vi "find start.vi"(6 "pulse sample":i32=5, 8 "trama length":i32=80, 9 "level":dbl=0.1 format="%#_13g", 10 "Trigger found in":bool, 11 "signal in":dbl[](array[numeric])) -> (2 "Trigger found":bool, 3 "signal out":dbl[](array[numeric]))   [LabVIEW 2017]
uses:
  <vilib>/Analysis/baseanly.llb/Real Dot Product.vi
  <vilib>/Analysis/NI_AAL_SigProc.lvlib
  <vilib>/Analysis/NI_AALBase.lvlib
panel:
  out "Numeric":dbl
  out "max index(es)":i32
  out "Waveform Graph":dbl[](graph)
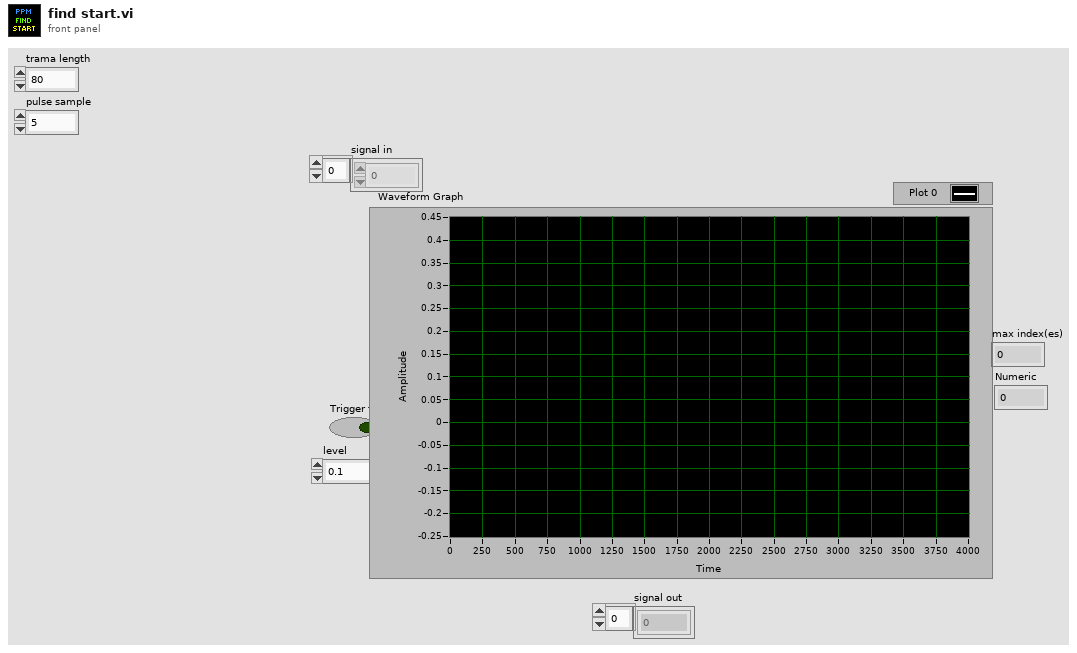
[diagram p1: front panel]
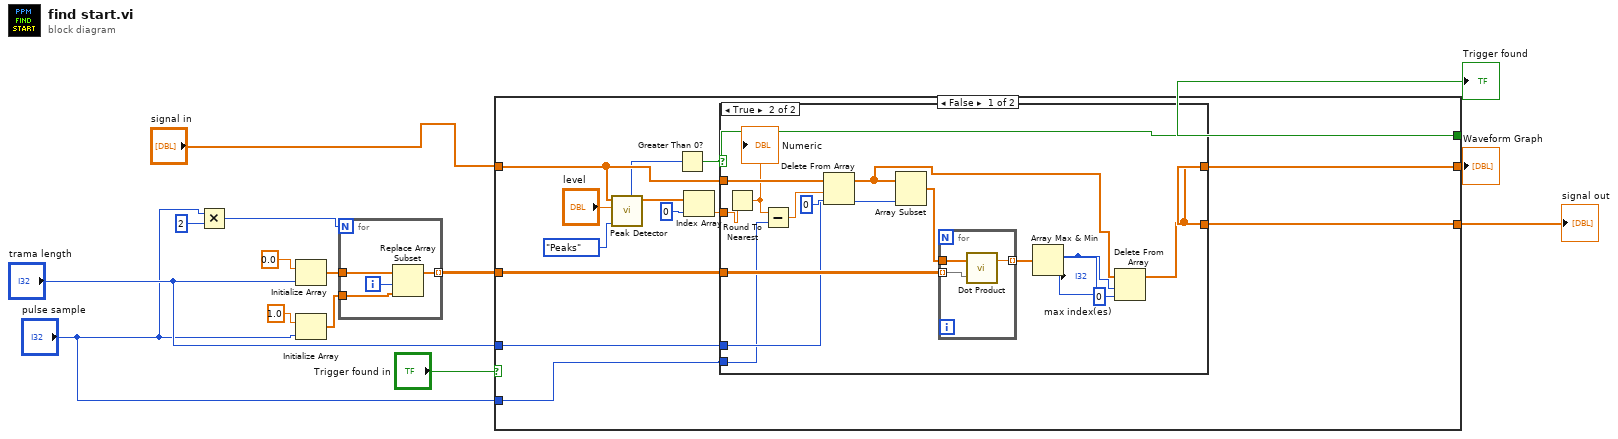
[diagram p0: block diagram]
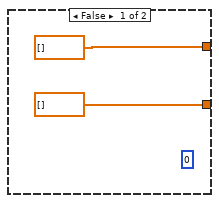
[diagram p2: hidden frame]
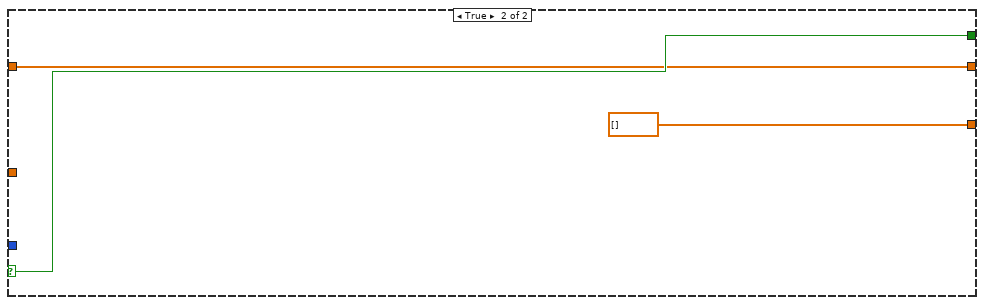
[diagram p3: hidden frame]
diagram:
  n1 = Multiply(x="pulse sample", y=u8 2) -> (x*y=w2:i32)
  n2 = Initialize Array(0.0 ("element"), "trama length") -> (w9:dbl[])
  n3 = Initialize Array(1.0 ("element"), "pulse sample") -> (w7:dbl[])
  n4 = for {
    N: w2 -> [_]
    tunnel: w9 -> [w17]
    tunnel: w7 -> [w16]
    tunnel: [w14] -> w6 mode=indexing
    i -> [w15]
    n5 = Replace Array Subset(array=w17, new element=w16, index=w15) -> (w14:dbl[])
  }
  n6 = case shown="False" "Trigger found in" {
    selector: "Trigger found in" -> [_ w52]
    tunnel: [w27 w52] -> w13
    tunnel: [w30 w51] -> w11
    tunnel: "signal in" -> [w28 w51]
    tunnel: [w20 dbl[] [] ("signal in")] -> _
    tunnel: w6 -> [w21 _]
    tunnel: "trama length" -> [w19 _]
    tunnel: "pulse sample" -> [w18 _]
    frame False {
      n7 = call <vilib>:"Peak Detector.vi"("peaks/valleys"=enum32{"Peaks", "Valleys"}."Peaks", "threshold"="level", "X"=w28) -> ("Locations"=w24:dbl[], "# found"=w26:i32)  [unwired: 4 in, 3 out]
      n8 = Greater Than 0?(x=w26) -> (x > 0?=w27:bool)
      n9 = Index Array(array=w24, index=0) -> (element=w23:dbl)
      n10 = case shown="True" w27 {
        tunnel: w28 -> [_ w46]
        tunnel: [dbl[] [] ("Y") w38] -> w30
        tunnel: w23 -> [_ w37]
        tunnel: [dbl[] [] ("signal in") w38] -> w20
        tunnel: w21 -> [_ w41]
        tunnel: w19 -> [_ w34]
        tunnel: w18 -> [_ w33]
        frame False {
          (unwired) 0
        }
        frame True {
          n11 = Round To Nearest(number=w37) -> (nearest integer value=w36:dbl)
          "Numeric" <- w36
          n12 = Subtract(x=w36, y=w33) -> (x-y=w44:dbl)
          n13 = Delete From Array(array=w46, length=w44, index=0) -> (array with subset deleted=w35:dbl[])  [unwired: 1 out]
          n14 = Array Subset(array=w35, length=w34) -> (w43:dbl[])  [unwired: 1 in]
          n15 = for {
            tunnel: w43 -> [w49]
            tunnel: [w48] -> w42 mode=indexing
            tunnel: w41 -> [w47] mode=indexing
            n16 = call-poly <vilib>:"Dot Product.vi"("Y Vector"=w47, "X Vector"=w49) -> ("X * Y"=w48:dbl)  [unwired: 1 out]
          }
          n17 = Array Max & Min(array=w42) -> (max index (indices)=w39:i32)  [unwired: 3 out]
          "max index(es)" <- w39
          n18 = Delete From Array(array=w35, length=w39, index=0) -> (array with subset deleted=w38:dbl[])  [unwired: 1 out]
        }
      }
    }
    frame True {
    }
  }
  "Trigger found" <- w13
  "signal out" <- w11
  "Waveform Graph" <- w11
